vi "Year2016_Question2.vi"() -> ()   [LabVIEW 2015]
panel:
  in  "stop":bool
  in  "Push Button":bool
  out "Counter":dbl
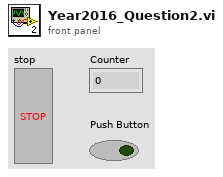
[diagram p1: front panel]
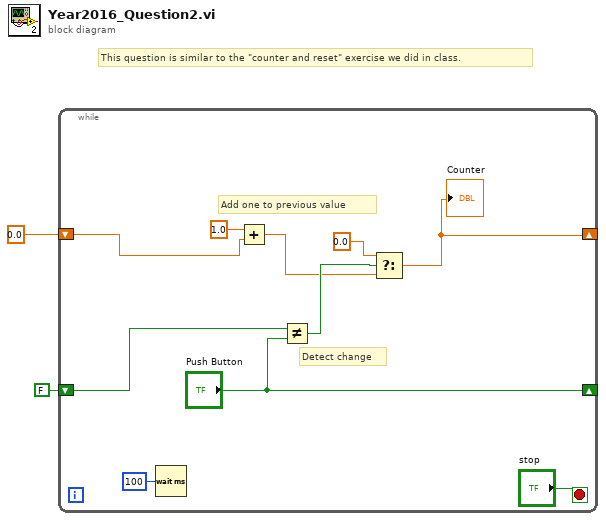
[diagram p0: block diagram]
diagram:
  # "This question is similar to the \"counter and reset\" exercise we did in class."
  n1 = while {
    shift-right: [w4] -> _
    shift-left: 0.0 -> [w11]
    shift-right: ["Push Button"] -> _
    shift-left: FALSE ("Push Button") -> [w9]
    stop <- "stop" stop-if-true
    # "Detect change"
    # "Add one to previous value"
    n2 = Wait (ms)(milliseconds to wait=u32 100) -> ()  [unwired: 1 out]
    n3 = Add(x=1.0, y=w11) -> (x+y=w5:dbl)
    n4 = Not Equal?(x=w9, y="Push Button") -> (x != y?=w7:bool)
    n5 = Select(t=0.0, s=w7, f=w5) -> (s? t:f=w4:dbl)
    "Counter" <- w4
  }
